vi "Pre Launch Init.vi"(11 "EDS Viewer in":refnum<class "EDS Viewer.lvclass">) -> (0 "error out":errorcluster, 3 "EDS Viewer out":refnum<class "EDS Viewer.lvclass">)   [LabVIEW 2024, in "EDS Viewer.lvlib" / "EDS Viewer.lvclass"]
doc: "Initializes the panel actor. Creates the Panel Helper.\n\n----\nPlease see the following web address for additional documentation and tutorial information:\nhttp://www.mooregoodideas.com/mgi-panel-manager/\n\nAuthor: Derek Trepanier\n\nCopyright (c) 2018, Moore Good Ideas, Inc.\n\nAll rights reserved.\n\nRedistribution and use in source and binary forms, with or without modification, are permitted provided that the following conditions are met:\n\n * Redistributions of source code must retain the above copyright notice, this list of conditions and the following disclaimer.\n * Redistributions in binary form must reproduce the above copyright notice, this list of conditions and the following disclaimer in the documentation and/or other materials provided with the distribution.\n * Neither the name of Moore Good Ideas, Inc. nor the names of its contributors may be used to endorse or promote products derived from this software without specific prior written permission.\n\nTHIS SOFTWARE IS PROVIDED BY THE COPYRIGHT HOLDERS AND CONTRIBUTORS \"AS IS\" AND ANY EXPRESS OR IMPLIED WARRANTIES, INCLUDING, BUT NOT LIMITED TO, THE IMPLIED WARRANTIES OF MERCHANTABILITY AND FITNESS FOR A PARTICULAR PURPOSE ARE DISCLAIMED. IN NO EVENT SHALL THE COPYRIGHT OWNER OR CONTRIBUTORS BE LIABLE FOR ANY DIRECT, INDIRECT, INCIDENTAL, SPECIAL, EXEMPLARY, OR CONSEQUENTIAL DAMAGES (INCLUDING, BUT NOT LIMITED TO, PROCUREMENT OF SUBSTITUTE GOODS OR SERVICES; LOSS OF USE, DATA, OR PROFITS; OR BUSINESS INTERRUPTION) HOWEVER CAUSED AND ON ANY THEORY OF LIABILITY, WHETHER IN CONTRACT, STRICT LIABILITY, OR TORT (INCLUDING NEGLIGENCE OR OTHERWISE) ARISING IN ANY WAY OUT OF THE USE OF THIS SOFTWARE, EVEN IF ADVISED OF THE POSSIBILITY OF SUCH DAMAGE."
uses:
  EDS Viewer.lvclass
  EDS Viewer.lvclass/EDS Viewer.ctl
  <vilib>/MGI/Panel Manager/Panel Actor/Panel Actor/Panel Actor.lvclass
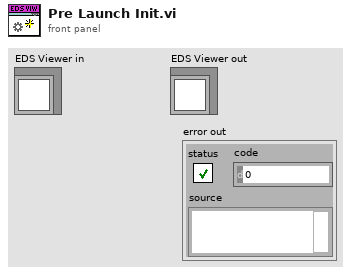
[diagram p1: front panel]
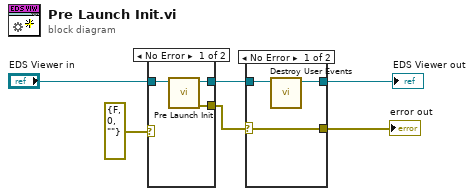
[diagram p0: block diagram]
diagram:
  n1 = case shown="No Error" errorcluster {"status"=FALSE, "code"=0, "source"=""} ("error IO") {
    selector: errorcluster {"status"=FALSE, "code"=0, "source"=""} ("error IO") -> [_ w11]
    tunnel: "EDS Viewer in" -> [w9 w10]
    tunnel: [w8 w10] -> w5
    tunnel: [w7 w11] -> w3
    frame No Error {
      n2 = call-parent "Pre Launch Init.vi"("Panel Actor in"=w9) -> ("error out"=w7:errorcluster, "Panel Actor out"=w8:refnum<class "EDS Viewer.lvclass">)  [unwired: 9 in]
    }
    frame Error {
    }
  }
  n3 = case shown="No Error" w3 {
    selector: w3 -> [w12 w15]
    tunnel: w5 -> [w14 w16]
    tunnel: [w13 w16] -> w4
    tunnel: [w12 w15] -> w2
    frame No Error {
      n4 = call-dynamic "Destroy User Events.vi"("EDS Viewer in"=w14) -> ("EDS Viewer out"=w13:refnum<class "EDS Viewer.lvclass">)  [unwired: 10 in]
    }
    frame Error {
    }
  }
  "error out" <- w2
  "EDS Viewer out" <- w4
